vi "Destroy user events.vi"(8 "error in (no error)":errorcluster, 11 "Signal_Gen in":refnum<class "Signal_Gen.lvclass">) -> (0 "error out":errorcluster, 3 "Signal_Gen out":refnum<class "Signal_Gen.lvclass">)   [LabVIEW 2019, in "Signal_Gen.lvlib" / "Signal_Gen.lvclass"]
uses:
  Signal_Gen.lvclass
  Signal_Gen.lvclass/Signal_Gen.ctl
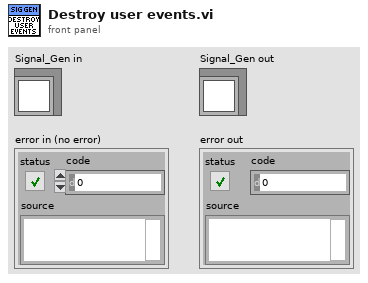
[diagram p1: front panel]
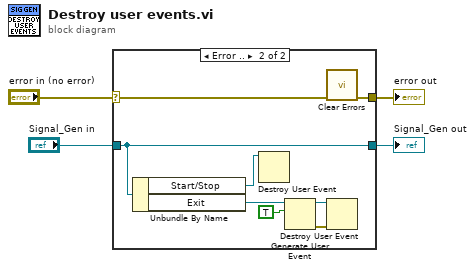
[diagram p0: block diagram]
diagram:
  n1 = case shown="Error .." "error in (no error)" {
    selector: "error in (no error)" -> [w6 w7]
    tunnel: [w6 w8] -> w2
    tunnel: [w5 w10] -> w3
    tunnel: "Signal_Gen in" -> [w5 w10]
    frame No Error {
    }
    frame Error {
      n2 = Unbundle By Name(w10) -> ("Start/Stop"=w11:refnum<user-event>, "Exit"=w12:refnum<user-event>)
      n3 = Destroy User Event(user event=w11) -> ()  [unwired: 1 in, 1 out]
      n4 = Generate User Event(user event=w12, event data cluster=TRUE ("event data")) -> (user event out=w14:refnum<user-event>, error out=w13:errorcluster)  [unwired: 2 in]
      n5 = call <vilib>:"Clear Errors.vi"("error in (no error)"=w7) -> ("error out"=w8:errorcluster)  [unwired: 5 in, 1 out]
      n6 = Destroy User Event(user event=w14, error in=w13) -> ()  [unwired: 1 out]
    }
  }
  "Signal_Gen out" <- w3
  "error out" <- w2
